vi "4.vi"() -> ()   [LabVIEW 2018]
panel:
  in  "stop":bool
  out "Boolean 2":bool
  in  "Boolean":bool
  out "Waveform Chart":dbl(graph)
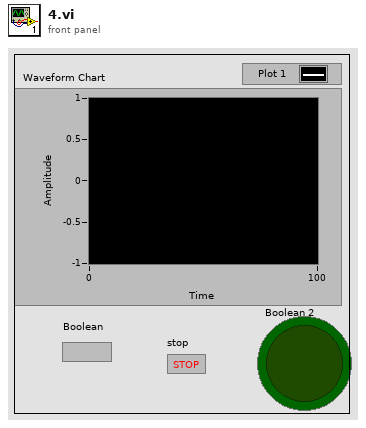
[diagram p1: front panel]
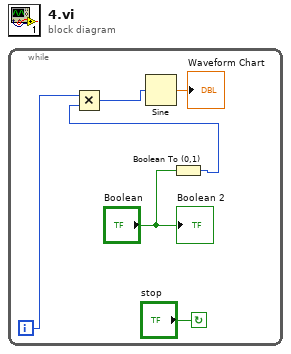
[diagram p0: block diagram]
diagram:
  n1 = while {
    i -> [w5]
    stop <- "stop" continue-if-true
    n2 = Boolean To (0,1)(Boolean="Boolean") -> (0, 1=w3:i16)
    n3 = Multiply(x=w5, y=w3) -> (x*y=w2:i32)
    n4 = Sine(x=w2) -> (sin(x)=→"Waveform Chart":dbl)
    "Boolean 2" <- "Boolean"
  }
